vi "Chirp module error reporter.vi"(8 "error in (no error)":errorcluster) -> ()   [LabVIEW 2017]
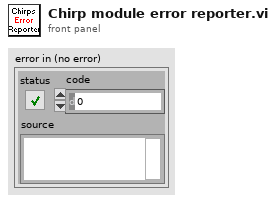
[diagram p1: front panel]
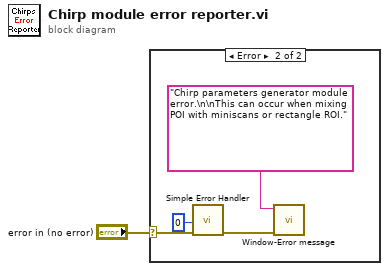
[diagram p0: block diagram]
diagram:
  n1 = case shown="Error" "error in (no error)" {
    selector: "error in (no error)" -> [_ w4]
    frame No Error {
    }
    frame Error {
      n2 = call <vilib>:"Simple Error Handler.vi"("type of dialog (OK msg:1)"=0, "error in (no error)"=w4) -> ("error out"=w2:errorcluster)  [unwired: 3 in, 4 out]
      n3 = call "Window-Error message.vi"("error in (no error)"=w2, "Message"="Chirp parameters generator module error.\n\nThis can occur when mixing POI with miniscans or rectangle ROI." ("format string")) -> ()  [unwired: 9 in, 1 out]
    }
  }
